vi "Process CAN State.vi"(8 "error in (no error)":errorcluster, 11 "State":T1 {"fault code" format="%08x"; "last error" items=["None", "Stuff", "Form", "Ack", "Bit1", "Bit0", "CRC"]; "communication state" items=["Error Active", "Error Passive", "Bus Off", "Init"]}) -> (0 "error out":errorcluster, 2 "Warning":bool, 3 "State":string)   [LabVIEW 2019, in "CAN Stream Support Workspace Shared.lvlib"]
uses:
  CAN Stream Support Workspace Shared.lvlib
  <vilib>/xnet/xnet.llb/XNET CAN Comm.ctl
  <vilib>/xnet/xnet.llb/XNET CAN Comm State.ctl
  <vilib>/xnet/xnet.llb/XNET CAN Last Err.ctl
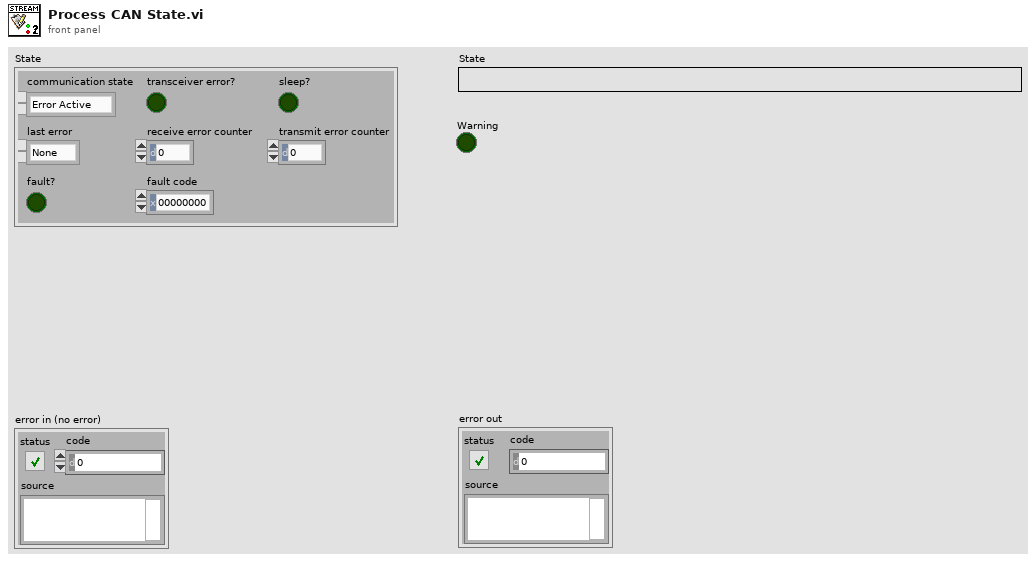
[diagram p1: front panel]
types:
  T1 = typedef "XNET CAN Comm.ctl" = cluster{"fault code":i32, "fault?":bool, "communication state":T2, "last error":T3, "receive error counter":u8, "transmit error counter":u8, "transceiver error?":bool, "sleep?":bool}
  T2 = typedef "XNET CAN Comm State.ctl" = u8
  T3 = typedef "XNET CAN Last Err.ctl" = u8
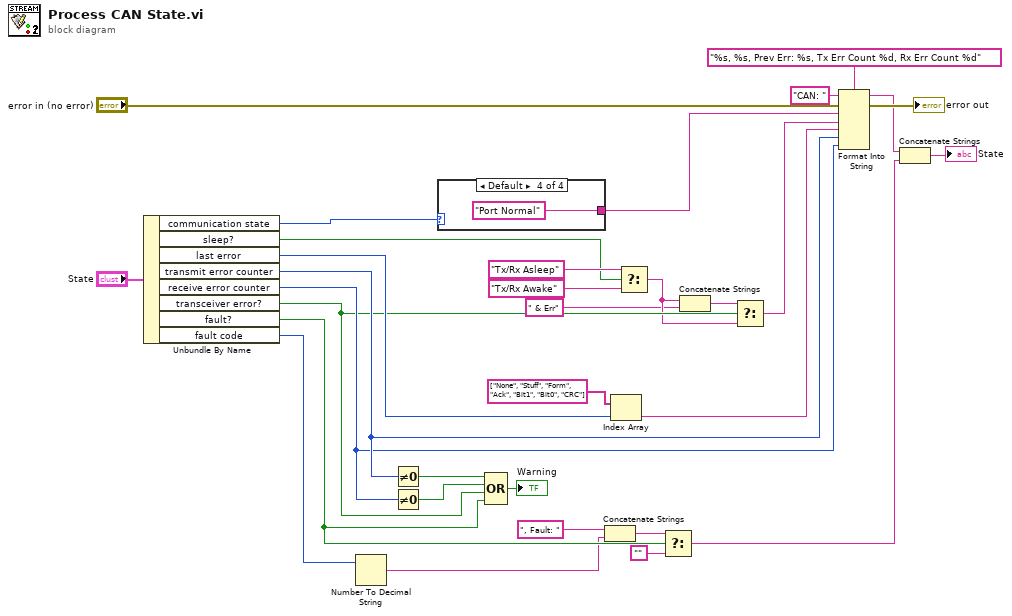
[diagram p0: block diagram]
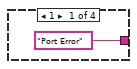
[diagram p2: hidden frame]
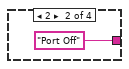
[diagram p3: hidden frame]
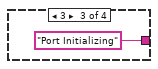
[diagram p4: hidden frame]
diagram:
  n1 = Unbundle By Name("State") -> ("communication state"=w25:T2, "sleep?"=w26:bool, "last error"=w22:T3, "transmit error counter"=w20:u8, "receive error counter"=w19:u8, "transceiver error?"=w14:bool, "fault?"=w13:bool, "fault code"=w12:i32)
  n2 = Number To Decimal String(number=w12) -> (decimal integer string=w10:string)  [unwired: 1 in]
  n3 = Not Equal To 0?(x=w20) -> (x != 0?=w17:bool)
  n4 = Not Equal To 0?(x=w19) -> (x != 0?=w18:bool)
  n5 = case shown="Default" w25 {
    tunnel: ["Port Error" "Port Off" "Port Initializing" "Port Normal"] -> w30
    frame 1 {
    }
    frame 2 {
    }
    frame 3 {
    }
    frame Default {
    }
  }
  n6 = Compound Arithmetic op=OR(w17, w18, w14, w13) -> (→"Warning":bool)
  n7 = Concatenate Strings(", Fault: " ("t"), w10) -> (w9:string)
  n8 = Index Array(array=string[] ["None", "Stuff", "Form", "Ack", "Bit1", "Bit0", "CRC"] ("Strings []"), index=w22) -> (element=w21:string)
  n9 = Select(t="Tx/Rx Asleep", s=w26, f="Tx/Rx Awake") -> (s? t:f=w4:string)
  n10 = Select(t=w9, s=w13, f="") -> (s? t:f=w5:string)
  n11 = Concatenate Strings(w4, " & Err" ("t")) -> (w2:string)
  n12 = Select(t=w2, s=w14, f=w4) -> (s? t:f=w15:string)
  n13 = Format Into String(format string="%s, %s, Prev Err: %s, Tx Err Count %d, Rx Err Count %d", initial string="CAN: ", error in="error in (no error)", w30, w15, w21, w20, w19) -> (resulting string=w7:string, error out=→"error out":errorcluster)
  n14 = Concatenate Strings(w7, w5) -> (→"State":string)
